vi "ziExample-ReadSingleValue.vi"(0 "Address":string="DEV", 1 "oscs/*/freq":dbl=12345.0 caption="Frequency (Hz)" format="%#_6p", 2 "demods/0/timeconstant":dbl=0.001 caption="TC (s)" format="%#_6p", 3 "phaseshift":dbl=12.0 caption="Phase (deg)" format="%#_6p", 4 "demods/0/harmonic":dbl caption="Harmonic", 5 "settingspath":string caption="Settings Path", 7 "Load":bool, 8 "Save":bool) -> (20 "Time since last boot (s)":dbl, 21 "R (Vrms)":dbl format="%#_4g", 22 "Theta (rad)":dbl, 24 "Selected Device":string)   [LabVIEW 2009]
doc: "Control a Zurich instrument device via the LabOne Labview API. \nRequirements: Zurich Instruments MFLI, HF2 or UHFLI \nExample from the Getting Started guide: A single demodulator value is read and unbundled read timestamp, X and Y.\n\n© Zurich Instruments AG, www.zhinst.com"
uses:
  <instrlib>/Zurich Instruments LabOne/Public/Data/ziTypeDemodSampleSingle.ctl
  <instrlib>/Zurich Instruments LabOne/Public/Utility/ziTicksToS_single.vi
  <instrlib>/Zurich Instruments LabOne/Public/Configure/ziGetValueDemodSampleEx.vi
  <instrlib>/Zurich Instruments LabOne/Public/Configure/ziSetValueDoubleArray.vi
  <instrlib>/Zurich Instruments LabOne/Public/Configure/ziGetValueDouble.vi
  <instrlib>/Zurich Instruments LabOne/Zurich Instruments LabOne.lvlib
panel:
  in  "stop":bool
  out "Demod Sample Out":T1={"Timestamps (ticks)"=0, "X (Vrms)"=nan, "Y (Vrms)"=nan, "Osc Phase (deg)"=nan, "Freq (Hz)"=nan, "DIO"=0, "AuxIn0 (V)"=nan, "AuxIn1 (V)"=nan, "Trigger"=0}
  out "Error Out":errorcluster
  # "This example describes how ziGetValueDemodSample.vi can be used"
  # "ziExample-ReadSingleValue.vi\nRequirements: HF2, UHFLI or MFLI\nsee block diagram for VI description"
  # "Settings"
  # "Unbundled output"
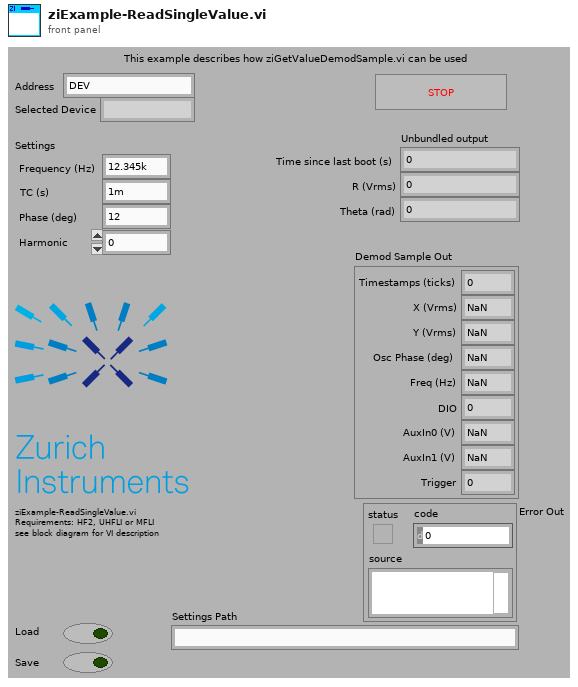
[diagram p1: front panel]
types:
  T1 = typedef "Zurich Instruments LabOne.lvlib/ziTypeDemodSampleSingle.ctl" = cluster{"Timestamps (ticks)":u64, "X (Vrms)":dbl, "Y (Vrms)":dbl, "Osc Phase (deg)":dbl, "Freq (Hz)":dbl, "DIO":u32, "AuxIn0 (V)":dbl, "AuxIn1 (V)":dbl, "Trigger":u32}
  T2 = typedef "Zurich Instruments LabOne.lvlib/ziTypeHandle.ctl" = cluster{"handleValid":bool, "Conn":u64, "Path Prefix":string, "Handle":u64, "Connected":bool, "Clockbase(s)":dbl}
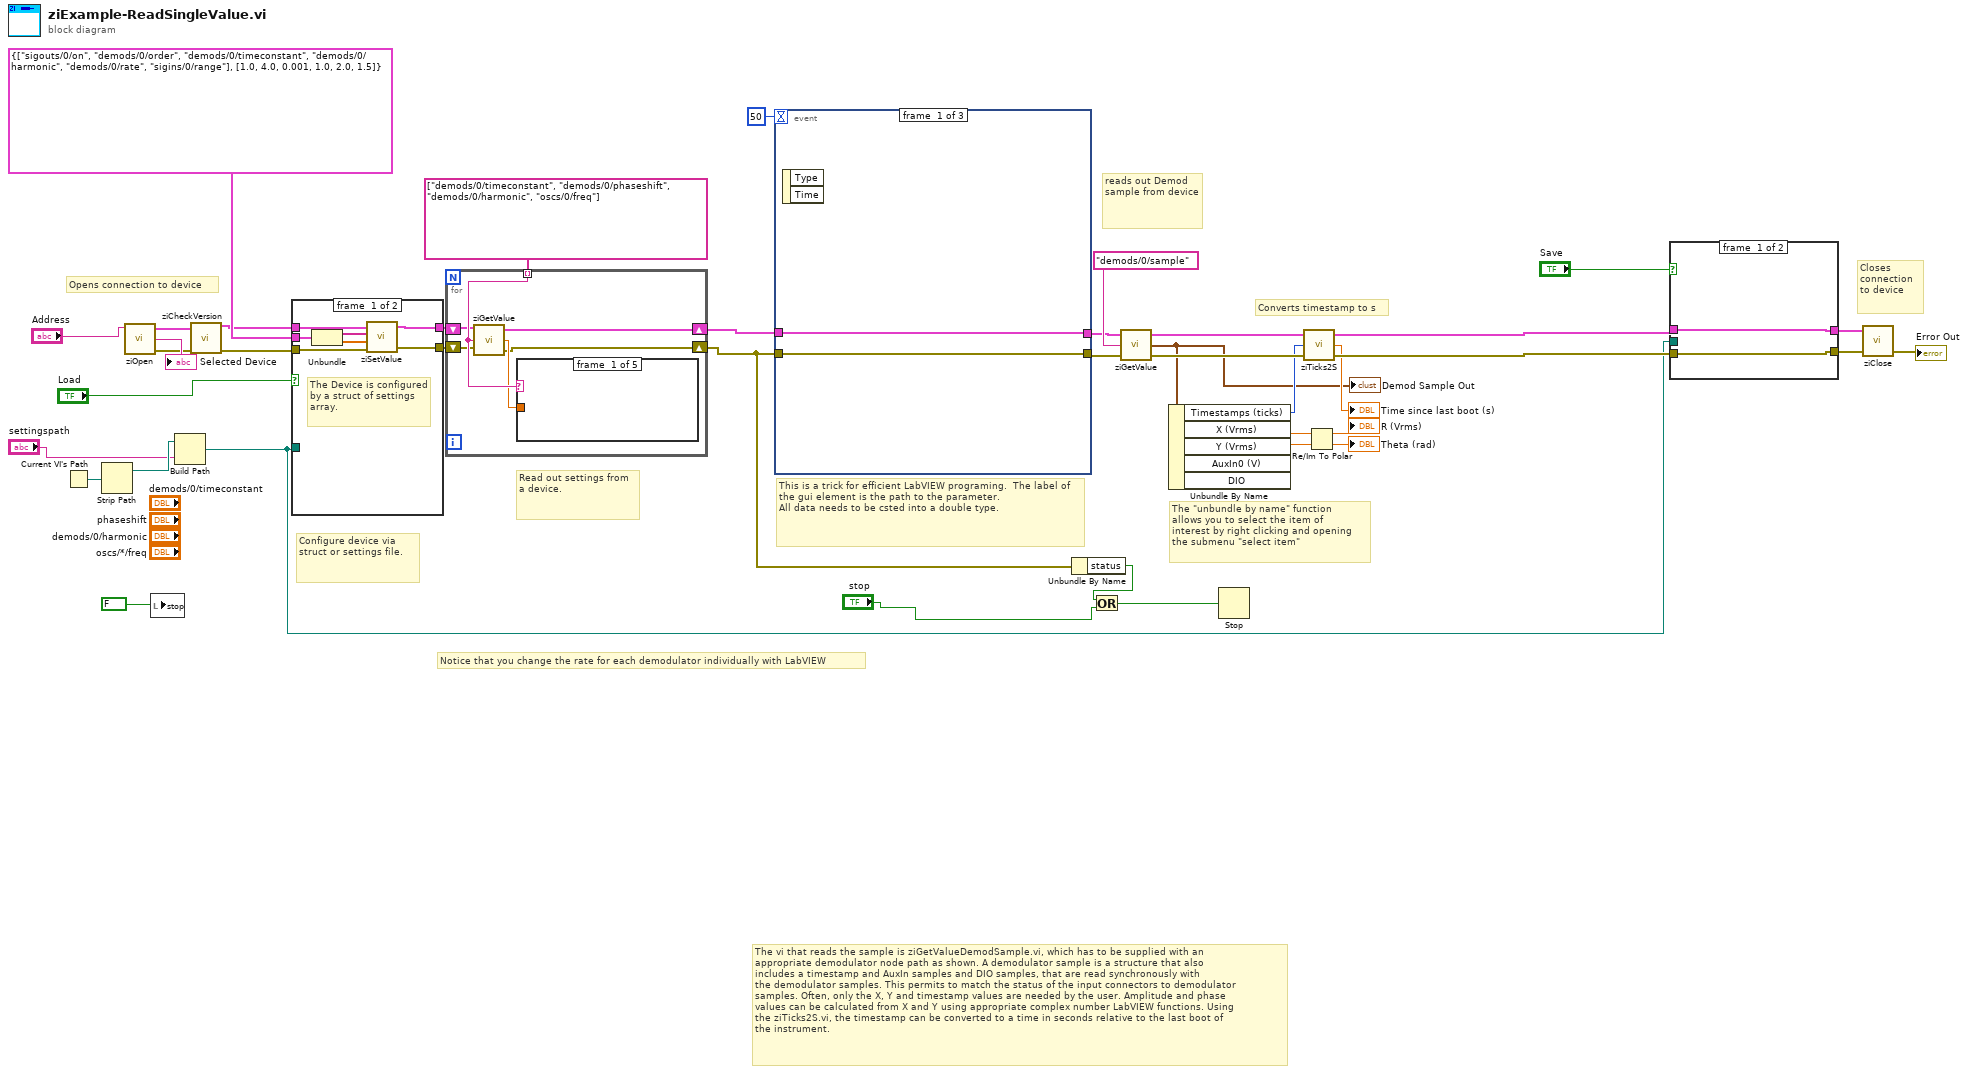
[diagram p0: block diagram]
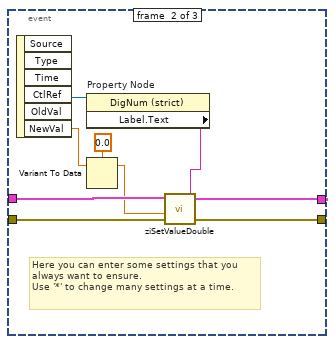
[diagram p2: hidden frame]
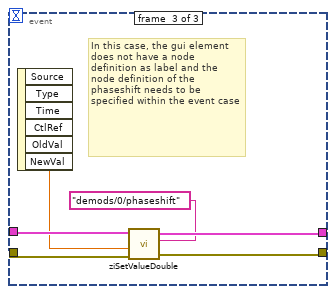
[diagram p3: hidden frame]
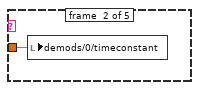
[diagram p4: hidden frame]
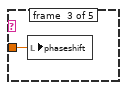
[diagram p5: hidden frame]
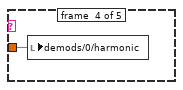
[diagram p6: hidden frame]
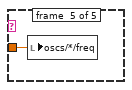
[diagram p7: hidden frame]
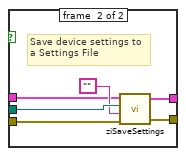
[diagram p8: hidden frame]
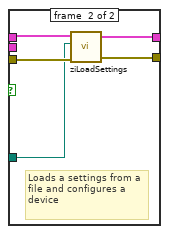
[diagram p9: hidden frame]
diagram:
  # "Converts timestamp to s"
  # "reads out Demod sample from device"
  # "This is a trick for efficient LabVIEW programing.  The label of the gui element is the path to the parameter.\nAll data needs to be csted into a double type."
  # "The \"unbundle by name\" function\nallows you to select the item of \ninterest by right clicking and opening\nthe submenu \"select item\""
  # "Closes connection to device"
  # "Opens connection to device"
  # "Read out settings from a device."
  # "Configure device via struct or settings file."
  # "Notice that you change the rate for each demodulator individually with LabVIEW"
  # "The vi that reads the sample is ziGetValueDemodSample.vi, which has to be supplied with an \nappropriate demodulator node path as shown. A demodulator sample is a structure that also \nincludes a timestamp and AuxIn samples and DIO samples, that are read synchronously with \nthe demodulator samples. This permits to match the status of the input connectors to demodulator \nsamples. Often, only the X, Y and timestamp values are needed by the user. Amplitude and phase\nvalues can be calculated from X and Y using appropriate complex number LabVIEW functions. Using \nthe ziTicks2S.vi, the timestamp can be converted to a time in seconds relative to the last boot of \nthe instrument."
  n1 = Current VI's Path() -> (path=w25:path)
  n2 = Strip Path(path=w25) -> (stripped path=w24:path)  [unwired: 1 out]
  n3 = call <instrlib>:"ziOpen.vi"("Address"="Address") -> ("Error Out"=w20:errorcluster, "Selected Device"=→"Selected Device":string, "HandleOut"=w21:T2)  [unwired: 3 in]
  n4 = local write "stop"(FALSE) -> ()
  n5 = Build Path(base path=w24, name or relative path="settingspath") -> (appended path=w22:path)
  n6 = call <instrlib>:"ziCheckVersion.vi"("Handle In"=w21, "Error In"=w20) -> ("Handle Out"=w18:T2, "Error Out"=w19:errorcluster)  [unwired: 11 in, 1 out]
  n7 = case shown="True" "Load" {
    tunnel: w19 -> [w47 w52]
    tunnel: w18 -> [w46 w49]
    tunnel: [w45 w50] -> w30
    tunnel: [w44 w51] -> w29
    tunnel: cluster{string[], dbl[]} {["sigouts/0/on", "demods/0/order", "demods/0/timeconstant", "demods/0/harmonic", "demods/0/rate", "sigins/0/range"], [1.0, 4.0, 0.001, 1.0, 2.0, 1.5]} -> [w43 _]
    tunnel: w22 -> [_ w48]
    frame #0 {
      # "The Device is configured by a struct of settings array."
      n8 = Unbundle(w43) -> (w42:string[], w41:dbl[])
      n9 = call-poly <instrlib>:"ziSetValue.vi"("Error In"=w47, "Values"=w41, "Paths"=w42, "Handle In"=w46) -> ("Error Out"=w44:errorcluster, "Handle Out"=w45:T2)  [unwired: 1 in]
    }
    frame #1 {
      # "Loads a settings from a file and configures a device"
      n10 = call <instrlib>:"ziLoadSettings.vi"("Error in"=w52, "File path (dialog if empty)"=w48, "Handle in"=w49) -> ("Error out"=w51:errorcluster, "Handle out"=w50:T2)  [unwired: 2 in]
    }
  }
  n11 = for {
    tunnel: string[] ["demods/0/timeconstant", "demods/0/phaseshift", "demods/0/harmonic", "oscs/0/freq"] -> [w58] mode=indexing
    shift-right: [w54] -> w28
    shift-left: w30 -> [w56]
    shift-right: [w53] -> w27
    shift-left: w29 -> [w55]
    n12 = call-poly <instrlib>:"ziGetValue.vi"("error in"=w55, "Path"=w58, "Handle in"=w56) -> ("error out"=w53:errorcluster, "Value"=w57:dbl, "Handle out"=w54:T2)
    n13 = case shown="\"demods/0/timeconstant\"" w58 {
      tunnel: w57 -> [_ w59 w60 w61 w62]
      frame #0 {
      }
      frame #1 {
        n14 = local write "demods/0/timeconstant"(w59) -> ()
      }
      frame #2 {
        n15 = local write "phaseshift"(w60) -> ()
      }
      frame #3 {
        n16 = local write "demods/0/harmonic"(w61) -> ()
      }
      frame #4 {
        n17 = local write "oscs/*/freq"(w62) -> ()
      }
    }
  }
  n18 = event shown="[1] \"oscs/*/freq\", \"demods/0/harmonic\", \"demods/0/timeconstant\": Value Change" {
    selector: _ -> [_ _ _]
    dyn-events: _ -> [_ _ _]
    timeout: 50 -> [_ _ _]
    tunnel: w28 -> [w64 w71 w78]
    tunnel: w27 -> [w63 w68 w77]
    tunnel: [w64 w70 w79] -> w4
    tunnel: [w63 w69 w76] -> w5
    event #0 {
      n19 = event-data() -> ()  [unwired: 3 out]
    }
    event #1 {
      # "Here you can enter some settings that you always want to ensure.\nUse '*' to change many settings at a time."
      n20 = event-data() -> ("CtlRef"=w73:refnum<vi>, "NewVal"=w72:dbl)  [unwired: 5 out]
      n21 = property on="Property Node" class="DigNum (strict)"(reference=w73) -> ("Label.Text"=w65:string)  [unwired: 1 in, 2 out]
      n22 = Variant To Data(Variant=w72, type=0.0 ("demods/")) -> (data=w67:dbl)  [unwired: 1 in, 1 out]
      n23 = call <instrlib>:"ziSetValueDouble.vi"("Error In"=w68, "Value"=w67, "Path"=w65, "Handle In"=w71) -> ("Error Out"=w69:errorcluster, "Handle Out"=w70:T2)  [unwired: 1 out]
    }
    event #2 {
      # "In this case, the gui element does not have a node definition as label and the node definition of the phaseshift needs to be\nspecified within the event case"
      n24 = event-data() -> ("NewVal"=w74:dbl)  [unwired: 6 out]
      n25 = call <instrlib>:"ziSetValueDouble.vi"("Error In"=w77, "Value"=w74, "Path"="demods/0/phaseshift", "Handle In"=w78) -> ("Error Out"=w76:errorcluster, "Handle Out"=w79:T2)  [unwired: 1 out]
    }
  }
  n26 = Unbundle By Name(w27) -> ("status"=w3:bool)
  n27 = Or(x=w3, y="stop") -> (x .or. y?=w1:bool)
  n28 = call-poly <instrlib>:"ziGetValue.vi"("error in"=w5, "Path"="demods/0/sample", "Handle In"=w4) -> ("error out"=w15:errorcluster, "Demod Sample Out"=w10:T1, "Handle Out"=w14:T2)
  "Demod Sample Out" <- w10
  n29 = Unbundle By Name(w10) -> ("Timestamps (ticks)"=w12:u64, "X (Vrms)"=w6:dbl, "Y (Vrms)"=w7:dbl)  [unwired: 2 out]
  n30 = Stop(stop? (T)=w1) -> ()
  n31 = call-poly <instrlib>:"ziTicks2S.vi"("Error In"=w15, "Timestamp(ticks)"=w12, "Handle In"=w14) -> ("Error Out"=w35:errorcluster, "Timestamp(s)"=→"Time since last boot (s)":dbl, "Handle Out"=w34:T2)
  n32 = Re/Im To Polar(2:w7, 3:w6) -> (0:→"Theta (rad)":dbl, 1:→"R (Vrms)":dbl)
  n33 = case shown="True" "Save" {
    tunnel: [w80 w86] -> w38
    tunnel: [w81 w85] -> w37
    tunnel: w22 -> [_ w87]
    tunnel: w35 -> [w81 w83]
    tunnel: w34 -> [w80 w82]
    frame #0 {
    }
    frame #1 {
      # "Save device settings to\na Settings File"
      n34 = call <instrlib>:"ziSaveSettings.vi"("Error In"=w83, "Path (\"\")"="", "file path (dialog if empty)"=w87, "Handle In"=w82) -> ("Error Out"=w85:errorcluster, "Handle Out"=w86:T2)  [unwired: 1 out]
    }
  }
  n35 = call <instrlib>:"ziClose.vi"("Error In"=w37, "Handle In"=w38) -> ("Error Out"=→"Error Out":errorcluster)  [unwired: 2 in, 1 out]
